vi "Read To File From Instrument.vi"(8 "error in (no error)":errorcluster, 9 "Target PC File":path=path "C:/test.wv", 10 "Source Instrument File":string="D:\\user\\data\\test.hcp", 11 "VISA resource name":refnum<visa-resource-name>) -> (0 "error out":errorcluster, 3 "VISA resource name out":refnum<visa-resource-name>)   [LabVIEW 2015, in "Rohde&Schwarz CMXP GPRF.lvlib"]
doc: "This VI copies a file from the instrument to the host computer:\n<b>INSTRUMENT FILE -> PC FILE</b>\n\nRemote-control command:\nMMEMory:DATA? '<file_name>'"
uses:
  <instrlib>/Rohde&Schwarz CMXP GPRF/Rohde&Schwarz CMXP GPRF.lvlib
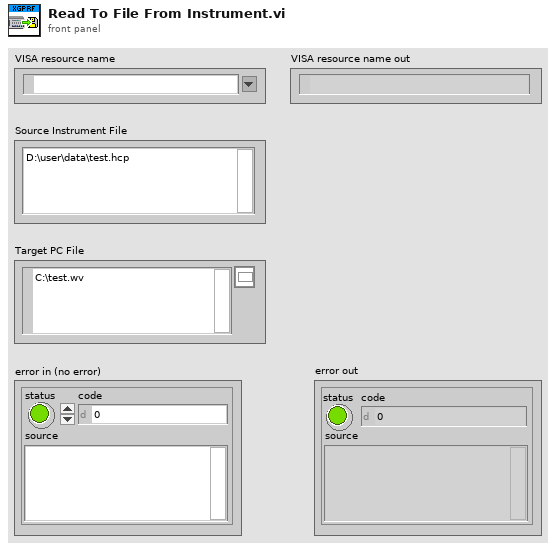
[diagram p1: front panel]
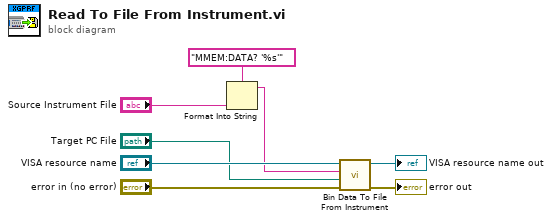
[diagram p0: block diagram]
diagram:
  n1 = Format Into String(format string="MMEM:DATA? '%s'", "Source Instrument File") -> (resulting string=w2:string)  [unwired: 2 in, 1 out]
  n2 = call <instrlib>:"Bin Data To File From Instrument.vi"("error in (no error)"="error in (no error)", "Target PC File"="Target PC File", "Query (\"\")"=w2, "VISA resource name"="VISA resource name") -> ("error out"=→"error out":errorcluster, "VISA resource name out"=→"VISA resource name out":refnum<visa-resource-name>)  [unwired: 6 in]
